vi "Write Image.vi"(8 "error in (no error)":errorcluster, 10 "Image":T1, 11 "Image Msg in":refnum<class "Image Msg.lvclass">) -> (0 "error out":errorcluster, 3 "Image Msg out":refnum<class "Image Msg.lvclass">)   [LabVIEW 2015, in "UI.lvlib" / "Image Msg.lvclass"]
uses:
  Image Msg.lvclass
  <vilib>/vision/Image Controls.llb/IMAQ Image.ctl
  Image Msg.lvclass/Image Msg.ctl
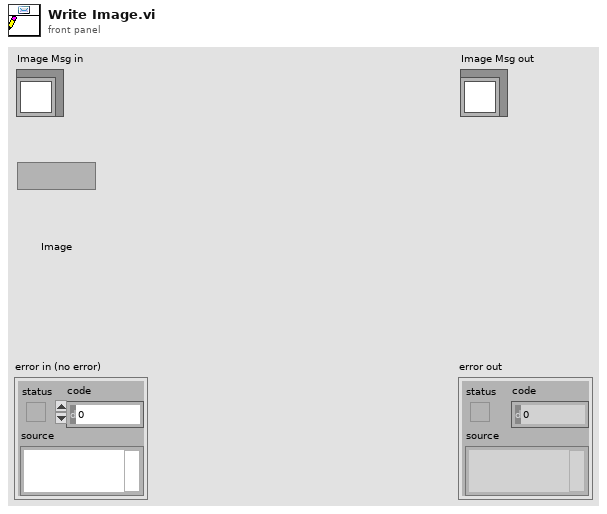
[diagram p1: front panel]
types:
  T1 = typedef "IMAQ Image.ctl" = refnum<image>
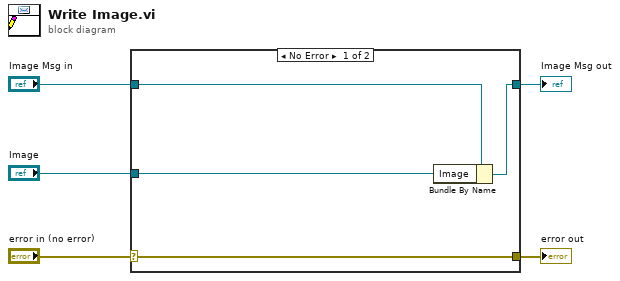
[diagram p0: block diagram]
diagram:
  n1 = case shown="No Error" "error in (no error)" {
    selector: "error in (no error)" -> [w9 w10]
    tunnel: [w9 w10] -> w4
    tunnel: [w7 w11] -> w2
    tunnel: "Image Msg in" -> [w8 w11]
    tunnel: "Image" -> [w6 _]
    frame No Error {
      n2 = Bundle By Name(cluster=w8, "Image"=w6) -> (w7:refnum<class "Image Msg.lvclass">)
    }
    frame Error {
    }
  }
  "error out" <- w4
  "Image Msg out" <- w2
